vi "mechanical_button.vi"() -> ()   [LabVIEW 2023]
panel:
  in  "Latch Until Released":bool
  out "led 6":bool
  out "Time (s)":dbl
  in  "Latch When Released":bool
  out "led 5":bool
  out "Time (s)":dbl
  in  "Latch When Pressed":bool
  out "led 4":bool
  out "Time (s)":dbl
  in  "Switch Until Released":bool
  out "led 3":bool
  out "Time (s)":dbl
  in  "Switch When Released":bool
  out "led 2":bool
  out "Time (s)":dbl
  in  "reset":bool
  out "Time (s)":dbl
  in  "stop":bool
  out "led":bool
  in  "Switch When Pressed":bool
  # "INSTRUCTIONS:"
  # "1) Press 'RESET' Button to reset the values of all the timers to zero\n2) Press \"STOP\" button to stop the program."
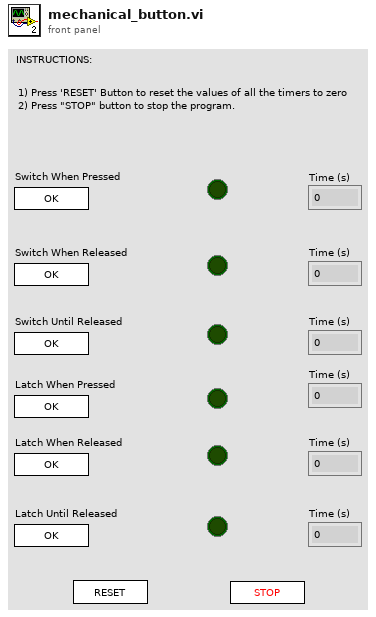
[diagram p1: front panel]
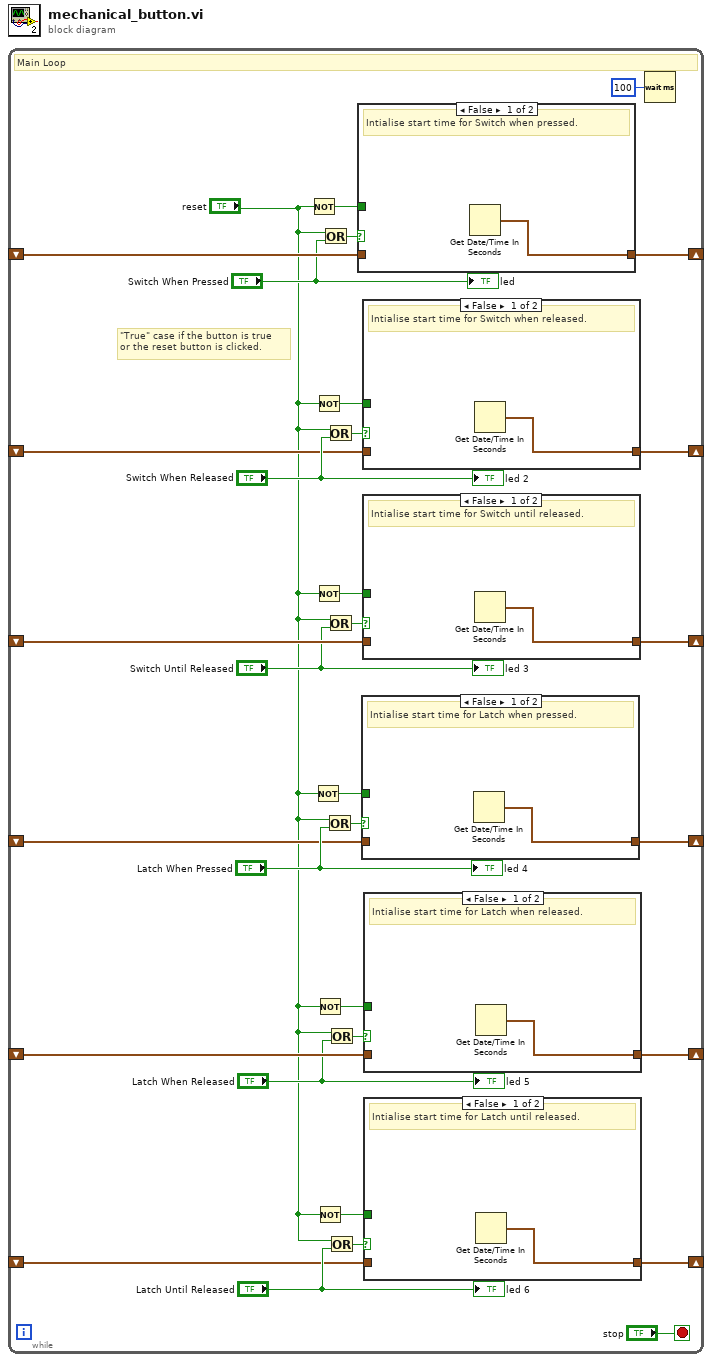
[diagram p0: block diagram]
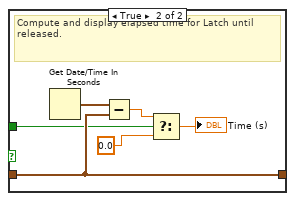
[diagram p2: hidden frame]
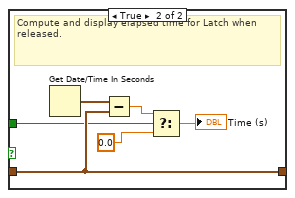
[diagram p3: hidden frame]
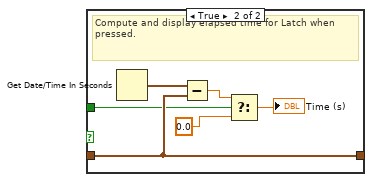
[diagram p4: hidden frame]
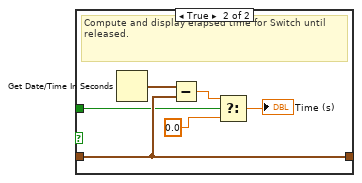
[diagram p5: hidden frame]
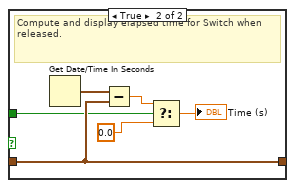
[diagram p6: hidden frame]
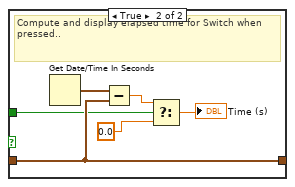
[diagram p7: hidden frame]
diagram:
  n1 = while {
    shift-right: [w31] -> _
    shift-left: _ -> [w30]
    shift-right: [w22] -> _
    shift-left: _ -> [w23]
    shift-right: [w21] -> _
    shift-left: _ -> [w20]
    shift-right: [w12] -> _
    shift-left: _ -> [w13]
    shift-right: [w11] -> _
    shift-left: _ -> [w10]
    shift-right: [w2] -> _
    shift-left: _ -> [w3]
    stop <- "stop" stop-if-true
    # "\"True\" case if the button is true \nor the reset button is clicked."
    # "Main Loop"
    n2 = Not(x="reset") -> (.not. x?=w29:bool)
    n3 = Not(x="reset") -> (.not. x?=w14:bool)
    n4 = Not(x="reset") -> (.not. x?=w24:bool)
    n5 = Not(x="reset") -> (.not. x?=w19:bool)
    n6 = Not(x="reset") -> (.not. x?=w9:bool)
    n7 = Not(x="reset") -> (.not. x?=w4:bool)
    n8 = Or(x="reset", y="Switch When Pressed") -> (x .or. y?=w27:bool)
    n9 = Or(x="reset", y="Latch When Pressed") -> (x .or. y?=w16:bool)
    n10 = Or(x="reset", y="Switch When Released") -> (x .or. y?=w26:bool)
    n11 = Or(x="reset", y="Switch Until Released") -> (x .or. y?=w17:bool)
    n12 = Or(x="reset", y="Latch When Released") -> (x .or. y?=w7:bool)
    n13 = Or(x="reset", y="Latch Until Released") -> (x .or. y?=w6:bool)
    n14 = case shown="False" w27 {
      tunnel: [w69 w73] -> w31
      tunnel: w30 -> [_ w73]
      tunnel: w29 -> [_ w70]
      frame False {
        # "Intialise start time for Switch when pressed."
        n15 = Get Date/Time In Seconds() -> (seconds since 1Jan1904=w69:timestamp)
      }
      frame True {
        # "Compute and display elapsed time for Switch when pressed.."
        n16 = Get Date/Time In Seconds() -> (seconds since 1Jan1904=w75:timestamp)
        n17 = Subtract(x=w75, y=w73) -> (x-y=w74:dbl)
        n18 = Select(t=w74, s=w70, f=0.0) -> (s? t:f=→"Time (s)":dbl)
      }
    }
    n19 = case shown="False" w16 {
      tunnel: [w48 w52] -> w12
      tunnel: w13 -> [_ w52]
      tunnel: w14 -> [_ w49]
      frame False {
        # "Intialise start time for Latch when pressed."
        n20 = Get Date/Time In Seconds() -> (seconds since 1Jan1904=w48:timestamp)
      }
      frame True {
        # "Compute and display elapsed time for Latch when pressed."
        n21 = Get Date/Time In Seconds() -> (seconds since 1Jan1904=w54:timestamp)
        n22 = Subtract(x=w54, y=w52) -> (x-y=w53:dbl)
        n23 = Select(t=w53, s=w49, f=0.0) -> (s? t:f=→"Time (s)":dbl)
      }
    }
    n24 = case shown="False" w26 {
      tunnel: [w62 w66] -> w22
      tunnel: w23 -> [_ w66]
      tunnel: w24 -> [_ w63]
      frame False {
        # "Intialise start time for Switch when released."
        n25 = Get Date/Time In Seconds() -> (seconds since 1Jan1904=w62:timestamp)
      }
      frame True {
        # "Compute and display elapsed time for Switch when released."
        n26 = Get Date/Time In Seconds() -> (seconds since 1Jan1904=w68:timestamp)
        n27 = Subtract(x=w68, y=w66) -> (x-y=w67:dbl)
        n28 = Select(t=w67, s=w63, f=0.0) -> (s? t:f=→"Time (s)":dbl)
      }
    }
    n29 = case shown="False" w17 {
      tunnel: [w55 w59] -> w21
      tunnel: w20 -> [_ w59]
      tunnel: w19 -> [_ w56]
      frame False {
        # "Intialise start time for Switch until released."
        n30 = Get Date/Time In Seconds() -> (seconds since 1Jan1904=w55:timestamp)
      }
      frame True {
        # "Compute and display elapsed time for Switch until released."
        n31 = Get Date/Time In Seconds() -> (seconds since 1Jan1904=w61:timestamp)
        n32 = Subtract(x=w61, y=w59) -> (x-y=w60:dbl)
        n33 = Select(t=w60, s=w56, f=0.0) -> (s? t:f=→"Time (s)":dbl)
      }
    }
    n34 = case shown="False" w7 {
      tunnel: [w41 w45] -> w11
      tunnel: w10 -> [_ w45]
      tunnel: w9 -> [_ w42]
      frame False {
        # "Intialise start time for Latch when released."
        n35 = Get Date/Time In Seconds() -> (seconds since 1Jan1904=w41:timestamp)
      }
      frame True {
        # "Compute and display elapsed time for Latch when released."
        n36 = Get Date/Time In Seconds() -> (seconds since 1Jan1904=w47:timestamp)
        n37 = Subtract(x=w47, y=w45) -> (x-y=w46:dbl)
        n38 = Select(t=w46, s=w42, f=0.0) -> (s? t:f=→"Time (s)":dbl)
      }
    }
    n39 = case shown="False" w6 {
      tunnel: [w34 w38] -> w2
      tunnel: w3 -> [_ w38]
      tunnel: w4 -> [_ w35]
      frame False {
        # "Intialise start time for Latch until released."
        n40 = Get Date/Time In Seconds() -> (seconds since 1Jan1904=w34:timestamp)
      }
      frame True {
        # "Compute and display elapsed time for Latch until released."
        n41 = Get Date/Time In Seconds() -> (seconds since 1Jan1904=w40:timestamp)
        n42 = Subtract(x=w40, y=w38) -> (x-y=w39:dbl)
        n43 = Select(t=w39, s=w35, f=0.0) -> (s? t:f=→"Time (s)":dbl)
      }
    }
    n44 = Wait (ms)(milliseconds to wait=u32 100) -> ()  [unwired: 1 out]
    "led" <- "Switch When Pressed"
    "led 2" <- "Switch When Released"
    "led 3" <- "Switch Until Released"
    "led 4" <- "Latch When Pressed"
    "led 5" <- "Latch When Released"
    "led 6" <- "Latch Until Released"
  }
